vi "Global_CMD to HW.vi"() -> ()   [LabVIEW 2017, in "Gear.lvlib"]
uses:
  Gear.lvlib
  ENUM_Servo Position.ctl
panel:
  in  "CMD Servo Positon":T1
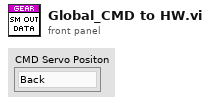
[diagram p1: front panel]
types:
  T1 = typedef "Gear.lvlib/ENUM_Servo Position.ctl" = enum16{"Back", "Forward"}
diagram:
